vi "yellow_street_vnutr.vi"() -> ()   [LabVIEW 2017]
uses:
  <vilib>/userdefined/High Color/IMAQdx.ctl
  <vilib>/myRIO/Instrument Drivers/Onboard IO/DIO/typedefs/DIO Reference.ctl
  <vilib>/myRIO/Common/Instrument Driver Framework/Utilities/typedefs/myRIO Generic Hardware Reference.ctl
  <vilib>/myRIO/Common/Instrument Driver Framework/Utilities/typedefs/Hardware Version Enum.ctl
  <vilib>/myRIO/Common/Instrument Driver Framework/Utilities/typedefs/myRIO v1.0 Reference.ctl
  <vilib>/myRIO/Common/Instrument Driver Framework/Utilities/typedefs/Generic FPGA Reference.ctl
  <vilib>/myRIO/Common/Instrument Driver Framework/myRIO v1.0/DIO/typedefs/DIO Channels List.ctl
  <vilib>/myRIO/Common/Instrument Driver Framework/myRIO v1.0/DIO/typedefs/DIO Channels Enum.ctl
  <vilib>/userdefined/High Color/nirio_resource_hc.ctl
  <vilib>/myRIO/Common/Instrument Driver Framework/Utilities/vis/Is FPGA Ref Available.vi
  <vilib>/myRIO/Common/Instrument Driver Framework/myRIO v1.0/DIO/vis/myRIO v1.1 Open DIO.vi
  <vilib>/myRIO/Instrument Drivers/Onboard IO/DIO/vis/Write.vi
  <vilib>/myRIO/Common/Instrument Driver Framework/Utilities/vis/Validate Channels.vi
  <vilib>/myRIO/Common/Instrument Driver Framework/myRIO v1.0/DIO/vis/myRIO v1.0 Reserve DIO.vi
  <vilib>/myRIO/Common/Instrument Driver Framework/myRIO v1.0/Resource Manager/vis/myRIO v1.0 Reserve Channel List.vi
  <vilib>/myRIO/Common/Instrument Driver Framework/myRIO v1.0/DIO/vis/myRIO v1.0 Build MUX Configuration DIO.vi
  <vilib>/myRIO/Common/Instrument Driver Framework/myRIO v1.0/Resource Manager/vis/myRIO v1.0 Reserve Channel.vi
  <vilib>/myRIO/Common/Instrument Driver Framework/myRIO v1.0/Resource Manager/vis/myRIO v1.0 Unreserve Channel.vi
  <vilib>/myRIO/Common/Instrument Driver Framework/myRIO v1.0/Resource Manager/vis/myRIO v1.0 Create Configuration List.vi
  <vilib>/myRIO/Common/Instrument Driver Framework/myRIO v1.0/Resource Manager/vis/myRIO v1.0 Build Mutex Name.vi
  <vilib>/Utility/VariantDataType/GetNumericInfo.vi
  <vilib>/Utility/error.llb/Error Cluster From Error Code.vi
  <vilib>/myRIO/Common/Instrument Driver Framework/myRIO v1.0/myRIO v1.1 Open.vi
  <vilib>/myRIO/Common/Instrument Driver Framework/Utilities/vis/IO Manager.vi
  <vilib>/myRIO/Common/Instrument Driver Framework/Utilities/vis/Configuration Manager.vi
  <vilib>/myRIO/Common/Instrument Driver Framework/myRIO v1.0/Resource Manager/vis/myRIO v1.0 Configure IO.vi
  <vilib>/myRIO/Common/Instrument Driver Framework/myRIO v1.0/myRIO v1.0 Close.vi
  <vilib>/myRIO/Common/Instrument Driver Framework/myRIO v1.0/DIO/vis/myRIO v1.0 Write DIO.vi
  <vilib>/myRIO/Express VI/Onboard Devices/LED/LED Express VI.xnode
  <vilib>/myRIO/Instrument Drivers/Onboard IO/DIO/vis/myRIO DIO Open.xnode
  <vilib>/vision/driver/NI_Vision_Acquisition_Software.lvlib
  <vilib>/myRIO/Instrument Drivers/Onboard IO/DIO/DIO.lvlib
panel:
  out "X 4":sgl
  out "X 3":sgl
  out "X 2":sgl
  out "X":sgl
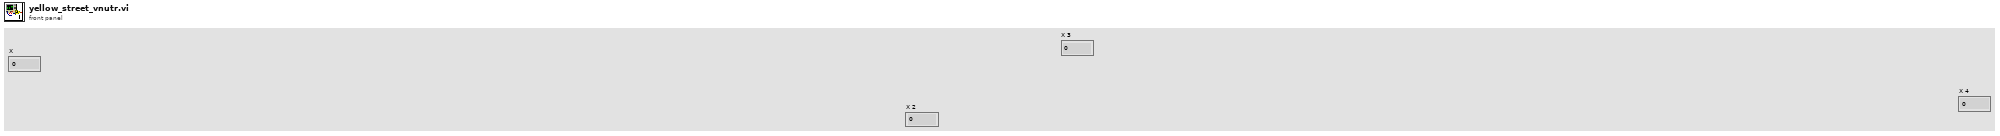
[diagram p1: front panel]
types:
  T1 = typedef "IMAQdx.ctl" = refnum<k21>
  T2 = typedef "DIO.lvlib/DIO Reference.ctl" = cluster{"myRIO Reference":T3, "DIO Channels List":T7}
  T3 = typedef "myRIO Generic Hardware Reference.ctl" = cluster{"myRIO Model":T4, "myRIO Hardware Reference":T5}
  T4 = typedef "Hardware Version Enum.ctl" = enum16{"Unknown", "myRIO-1900", "myRIO-1950", "roboRIO", "NI ELVIS RIO CM"}
  T5 = typedef "myRIO v1.0 Reference.ctl" = cluster{"Generic FPGA Reference":T6, "Allow multiple opens":bool}
  T6 = typedef "Generic FPGA Reference.ctl" = refnum<k20>
  T7 = typedef "DIO Channels List.ctl" = T8[]
  T8 = typedef "DIO Channels Enum.ctl" = enum16{"Not Connected", "C/DIO0", "C/DIO1", "C/DIO2", "C/DIO3", "C/DIO4", "C/DIO5", "C/DIO6", "C/DIO7", "A/DIO0", "A/DIO1", "A/DIO2", "A/DIO3", "A/DIO4", "A/DIO5", "A/DIO6", "A/DIO7", "A/DIO8", "A/DIO9", "A/DIO10", "A/DIO11", "A/DIO12", "A/DIO13", "A/DIO14", "A/DIO15", "B/DIO0", "B/DIO1", "B/DIO2", "B/DIO3", "B/DIO4", "B/DIO5", "B/DIO6", "B/DIO7", "B/DIO8", "B/DIO9", "B/DIO10", "B/DIO11", "B/DIO12", "B/DIO13", "B/DIO14", "B/DIO15", "LED0", "LED1", "LED2", "LED3", "Button0", "DIO/DIO0", "DIO/DIO1", "DIO/DIO2", "DIO/DIO3", "DIO/DIO4", "DIO/DIO5", "DIO/DIO6", "DIO/DIO7", "DIO/DIO8", "DIO/DIO9", "SPI/CS0", "SPI/CS1", "SPI/CS2", "SPI/CS3", "LED RADIO (Green)", "LED RADIO (Red)", "LED COMM (Green)", "LED COMM (Red)", "LED MODE (Green)", "LED MODE (Red)"}
  T9 = typedef "nirio_resource_hc.ctl" = tag
  T10 = typedef "IMAQ Image.ctl" = refnum<image>
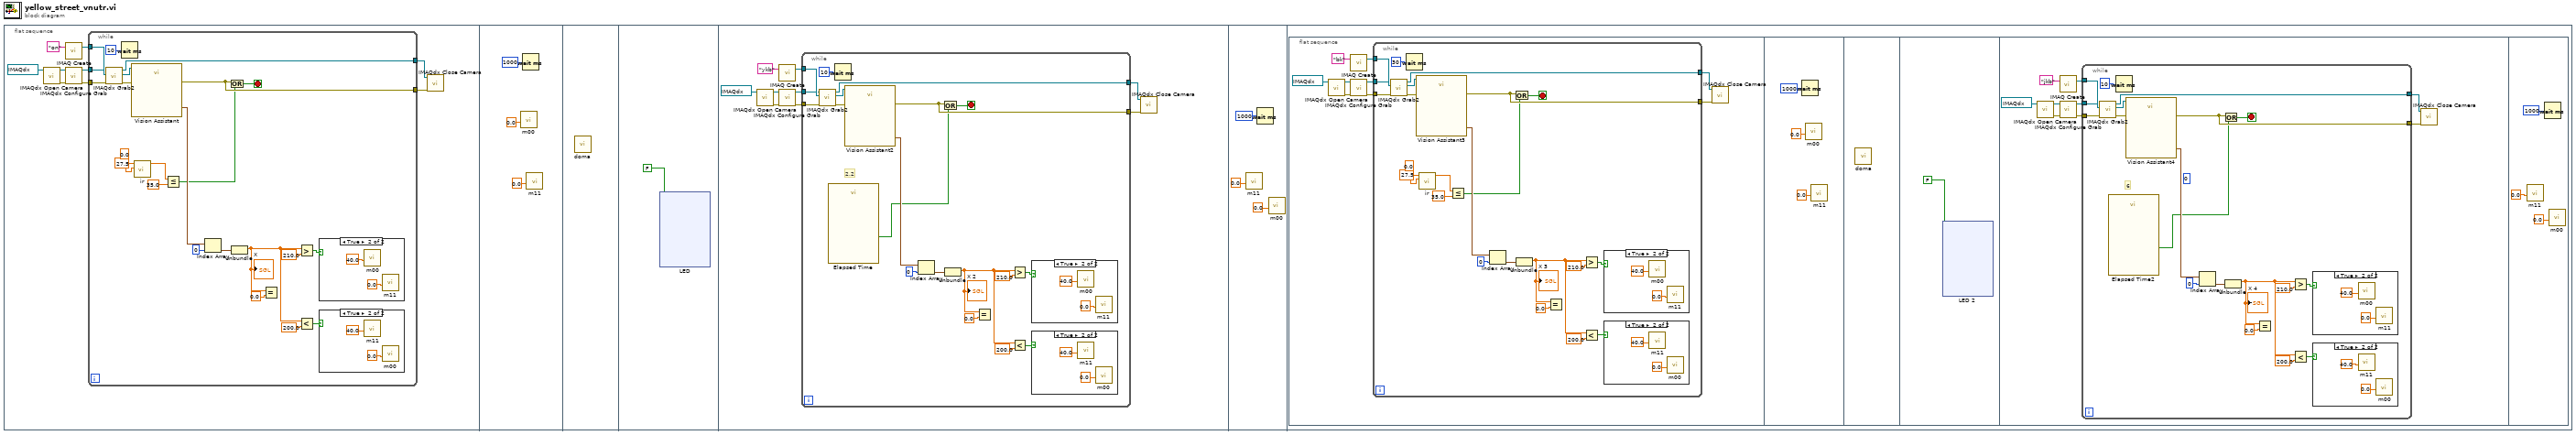
[diagram p0: block diagram]
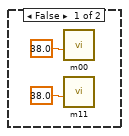
[diagram p2: hidden frame]
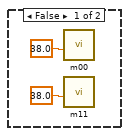
[diagram p3: hidden frame]
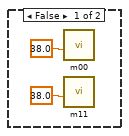
[diagram p4: hidden frame]
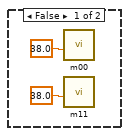
[diagram p5: hidden frame]
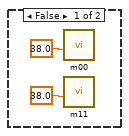
[diagram p6: hidden frame]
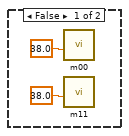
[diagram p7: hidden frame]
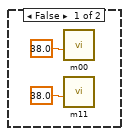
[diagram p8: hidden frame]
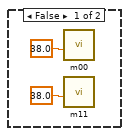
[diagram p9: hidden frame]
diagram:
  n1 = flat-sequence {
    frame #0 {
      n2 = call <vilib>:"IMAQdx Open Camera.vi"("Session In"=T1 "cam1") -> ("error out"=w6:errorcluster, "Session Out"=w5:T1)  [unwired: 9 in]
      n3 = call "IMAQ Create"("Image Name"="on") -> ("New Image"=w3:T10)  [unwired: 4 in, 1 out]
      n4 = call <vilib>:"IMAQdx Configure Grab.vi"("error in"=w6, "Session In"=w5) -> ("error out"=w7:errorcluster, "Session Out"=w4:T1)  [unwired: 8 in]
      n5 = while {
        tunnel: w7 -> [w27]
        tunnel: w3 -> [w26]
        tunnel: w4 -> [w25]
        tunnel: [w24] -> w9
        tunnel: [w23] -> w8
        stop <- w10 stop-if-true
        n6 = call <vilib>:"IMAQdx Grab2.vi"("error in"=w27, "Image In"=w26, "Session In"=w25) -> ("error out"=w29:errorcluster, "Image Out"=w28:T10, "Session Out"=w24:T1)  [unwired: 5 in, 1 out]
        n7 = Wait (ms)(milliseconds to wait=u32 10) -> ()  [unwired: 1 out]
        n8 = call "Vision Assistant"("Image In"=w28, "error in"=w29) -> ("Edges Coordinates (Edge Detector 1)"=w32:cluster{"X":sgl, "Y":sgl}[], "error out"=w23:errorcluster)  [unwired: 22 in, 2 out]
        n9 = call "ir.vi"("Koffset [cm]"=0.0, "Kscale [cm-V]"=27.5) -> ("см"=w15:dbl)  [unwired: 8 in, 1 out]
        n10 = Less Or Equal?(x=w15, y=35.0) -> (x <= y?=w11:bool)
        n11 = Index Array(array=w32, index=0) -> (element=w31:cluster{"X":sgl, "Y":sgl})
        n12 = Or(x=w23, y=w11) -> (x .or. y?=w10:bool)
        n13 = Unbundle(w31) -> ("X"=w18:sgl)  [unwired: 1 out]
        "X" <- w18
        n14 = Equal?(x=w18, y=sgl 0.0) -> ()  [unwired: 1 out]
        n15 = Greater?(x=w18, y=sgl 210.0) -> (0:w21:bool)
        n16 = Less?(x=w18, y=sgl 200.0) -> (x < y?=w17:bool)
        n17 = case shown="True" w21 {
          frame False {
            n18 = call "m00.vi"("position"=38.0) -> ()  [unwired: 10 in, 1 out]
            n19 = call "m11.vi"("position"=38.0) -> ()  [unwired: 10 in, 1 out]
          }
          frame True {
            n20 = call "m00.vi"("position"=40.0) -> ()  [unwired: 10 in, 1 out]
            n21 = call "m11.vi"("position"=0.0) -> ()  [unwired: 10 in, 1 out]
          }
        }
        n22 = case shown="True" w17 {
          frame False {
            n23 = call "m00.vi"("position"=38.0) -> ()  [unwired: 10 in, 1 out]
            n24 = call "m11.vi"("position"=38.0) -> ()  [unwired: 10 in, 1 out]
          }
          frame True {
            n25 = call "m11.vi"("position"=40.0) -> ()  [unwired: 10 in, 1 out]
            n26 = call "m00.vi"("position"=0.0) -> ()  [unwired: 10 in, 1 out]
          }
        }
      }
      n27 = call <vilib>:"IMAQdx Close Camera.vi"("error in"=w8, "Session In"=w9) -> ()  [unwired: 9 in, 1 out]
    }
    frame #1 {
      n28 = call "m00.vi"("position"=0.0) -> ()  [unwired: 10 in, 1 out]
      n29 = Wait (ms)(milliseconds to wait=u32 1000) -> ()  [unwired: 1 out]
      n30 = call "m11.vi"("position"=0.0) -> ()  [unwired: 10 in, 1 out]
    }
    frame #2 {
      n31 = call "doma.vi"() -> ()  [unwired: 12 in]
    }
    frame #3 {
      w44 = FALSE
      n32 = xnode "LED"("LED0"=w44, "LED1"=w44, "LED2"=w44, "LED3"=w44) -> ()  [unwired: 1 in, 1 out]
    }
    frame #4 {
      n33 = call <vilib>:"IMAQdx Open Camera.vi"("Session In"=T1 "cam1") -> ("error out"=w88:errorcluster, "Session Out"=w87:T1)  [unwired: 9 in]
      n34 = call "IMAQ Create"("Image Name"="ykb") -> ("New Image"=w85:T10)  [unwired: 4 in, 1 out]
      n35 = call <vilib>:"IMAQdx Configure Grab.vi"("error in"=w88, "Session In"=w87) -> ("error out"=w89:errorcluster, "Session Out"=w86:T1)  [unwired: 8 in]
      n36 = while {
        tunnel: w89 -> [w105]
        tunnel: w85 -> [w104]
        tunnel: w86 -> [w103]
        tunnel: [w102] -> w91
        tunnel: [w101] -> w90
        stop <- w93 stop-if-true
        # "2,2"
        n37 = call <vilib>:"IMAQdx Grab2.vi"("error in"=w105, "Image In"=w104, "Session In"=w103) -> ("error out"=w107:errorcluster, "Image Out"=w106:T10, "Session Out"=w102:T1)  [unwired: 5 in, 1 out]
        n38 = call "Elapsed Time"() -> ("Time has Elapsed"=w92:bool)  [unwired: 12 in, 7 out]
        n39 = Wait (ms)(milliseconds to wait=u32 10) -> ()  [unwired: 1 out]
        n40 = call "Vision Assistant2"("Image In"=w106, "error in"=w107) -> ("Edges Coordinates (Edge Detector 1)"=w110:cluster{"X":sgl, "Y":sgl}[], "error out"=w101:errorcluster)  [unwired: 22 in, 2 out]
        n41 = Index Array(array=w110, index=0) -> (element=w109:cluster{"X":sgl, "Y":sgl})
        n42 = Or(x=w101, y=w92) -> (x .or. y?=w93:bool)
        n43 = Unbundle(w109) -> ("X"=w96:sgl)  [unwired: 1 out]
        "X 2" <- w96
        n44 = Equal?(x=w96, y=sgl 0.0) -> ()  [unwired: 1 out]
        n45 = Greater?(x=w96, y=sgl 210.0) -> (0:w99:bool)
        n46 = Less?(x=w96, y=sgl 200.0) -> (x < y?=w95:bool)
        n47 = case shown="True" w99 {
          frame False {
            n48 = call "m00.vi"("position"=38.0) -> ()  [unwired: 10 in, 1 out]
            n49 = call "m11.vi"("position"=38.0) -> ()  [unwired: 10 in, 1 out]
          }
          frame True {
            n50 = call "m00.vi"("position"=40.0) -> ()  [unwired: 10 in, 1 out]
            n51 = call "m11.vi"("position"=0.0) -> ()  [unwired: 10 in, 1 out]
          }
        }
        n52 = case shown="True" w95 {
          frame False {
            n53 = call "m00.vi"("position"=38.0) -> ()  [unwired: 10 in, 1 out]
            n54 = call "m11.vi"("position"=38.0) -> ()  [unwired: 10 in, 1 out]
          }
          frame True {
            n55 = call "m11.vi"("position"=40.0) -> ()  [unwired: 10 in, 1 out]
            n56 = call "m00.vi"("position"=0.0) -> ()  [unwired: 10 in, 1 out]
          }
        }
      }
      n57 = call <vilib>:"IMAQdx Close Camera.vi"("error in"=w90, "Session In"=w91) -> ()  [unwired: 9 in, 1 out]
    }
    frame #5 {
      n58 = call "m11.vi"("position"=0.0) -> ()  [unwired: 10 in, 1 out]
      n59 = Wait (ms)(milliseconds to wait=u32 1000) -> ()  [unwired: 1 out]
      n60 = call "m00.vi"("position"=0.0) -> ()  [unwired: 10 in, 1 out]
    }
    frame #6 {
      n61 = flat-sequence {
        frame #0 {
          n62 = call <vilib>:"IMAQdx Open Camera.vi"("Session In"=T1 "cam1") -> ("error out"=w127:errorcluster, "Session Out"=w126:T1)  [unwired: 9 in]
          n63 = call "IMAQ Create"("Image Name"="bk") -> ("New Image"=w124:T10)  [unwired: 4 in, 1 out]
          n64 = call <vilib>:"IMAQdx Configure Grab.vi"("error in"=w127, "Session In"=w126) -> ("error out"=w128:errorcluster, "Session Out"=w125:T1)  [unwired: 8 in]
          n65 = while {
            tunnel: w128 -> [w148]
            tunnel: w124 -> [w147]
            tunnel: w125 -> [w146]
            tunnel: [w145] -> w130
            tunnel: [w144] -> w129
            stop <- w131 stop-if-true
            n66 = call <vilib>:"IMAQdx Grab2.vi"("error in"=w148, "Image In"=w147, "Session In"=w146) -> ("error out"=w150:errorcluster, "Image Out"=w149:T10, "Session Out"=w145:T1)  [unwired: 5 in, 1 out]
            n67 = Wait (ms)(milliseconds to wait=u32 30) -> ()  [unwired: 1 out]
            n68 = call "Vision Assistant3"("Image In"=w149, "error in"=w150) -> ("Edges Coordinates (Edge Detector 1)"=w153:cluster{"X":sgl, "Y":sgl}[], "error out"=w144:errorcluster)  [unwired: 22 in, 2 out]
            n69 = call "ir.vi"("Koffset [cm]"=0.0, "Kscale [cm-V]"=27.5) -> ("см"=w136:dbl)  [unwired: 8 in, 1 out]
            n70 = Less Or Equal?(x=w136, y=35.0) -> (x <= y?=w132:bool)
            n71 = Index Array(array=w153, index=0) -> (element=w152:cluster{"X":sgl, "Y":sgl})
            n72 = Or(x=w144, y=w132) -> (x .or. y?=w131:bool)
            n73 = Unbundle(w152) -> ("X"=w139:sgl)  [unwired: 1 out]
            "X 3" <- w139
            n74 = Equal?(x=w139, y=sgl 0.0) -> ()  [unwired: 1 out]
            n75 = Greater?(x=w139, y=sgl 210.0) -> (0:w142:bool)
            n76 = Less?(x=w139, y=sgl 200.0) -> (x < y?=w138:bool)
            n77 = case shown="True" w142 {
              frame False {
                n78 = call "m00.vi"("position"=38.0) -> ()  [unwired: 10 in, 1 out]
                n79 = call "m11.vi"("position"=38.0) -> ()  [unwired: 10 in, 1 out]
              }
              frame True {
                n80 = call "m00.vi"("position"=40.0) -> ()  [unwired: 10 in, 1 out]
                n81 = call "m11.vi"("position"=0.0) -> ()  [unwired: 10 in, 1 out]
              }
            }
            n82 = case shown="True" w138 {
              frame False {
                n83 = call "m00.vi"("position"=38.0) -> ()  [unwired: 10 in, 1 out]
                n84 = call "m11.vi"("position"=38.0) -> ()  [unwired: 10 in, 1 out]
              }
              frame True {
                n85 = call "m11.vi"("position"=40.0) -> ()  [unwired: 10 in, 1 out]
                n86 = call "m00.vi"("position"=0.0) -> ()  [unwired: 10 in, 1 out]
              }
            }
          }
          n87 = call <vilib>:"IMAQdx Close Camera.vi"("error in"=w129, "Session In"=w130) -> ()  [unwired: 9 in, 1 out]
        }
        frame #1 {
          n88 = Wait (ms)(milliseconds to wait=u32 1000) -> ()  [unwired: 1 out]
          n89 = call "m00.vi"("position"=0.0) -> ()  [unwired: 10 in, 1 out]
          n90 = call "m11.vi"("position"=0.0) -> ()  [unwired: 10 in, 1 out]
        }
        frame #2 {
          n91 = call "doma.vi"() -> ()  [unwired: 12 in]
        }
        frame #3 {
          w165 = FALSE
          n92 = xnode "LED 2"("LED0"=w165, "LED1"=w165, "LED2"=w165, "LED3"=w165) -> ()  [unwired: 1 in, 1 out]
        }
        frame #4 {
          n93 = call <vilib>:"IMAQdx Open Camera.vi"("Session In"=T1 "cam1") -> ("error out"=w209:errorcluster, "Session Out"=w208:T1)  [unwired: 9 in]
          n94 = call "IMAQ Create"("Image Name"="jkb") -> ("New Image"=w206:T10)  [unwired: 4 in, 1 out]
          n95 = call <vilib>:"IMAQdx Configure Grab.vi"("error in"=w209, "Session In"=w208) -> ("error out"=w210:errorcluster, "Session Out"=w207:T1)  [unwired: 8 in]
          n96 = while {
            tunnel: w210 -> [w226]
            tunnel: w206 -> [w225]
            tunnel: w207 -> [w224]
            tunnel: [w223] -> w212
            tunnel: [w222] -> w211
            stop <- w214 stop-if-true
            (unwired) 0 ("index")
            # "6"
            n97 = call <vilib>:"IMAQdx Grab2.vi"("error in"=w226, "Image In"=w225, "Session In"=w224) -> ("error out"=w228:errorcluster, "Image Out"=w227:T10, "Session Out"=w223:T1)  [unwired: 5 in, 1 out]
            n98 = call "Elapsed Time2"() -> ("Time has Elapsed"=w213:bool)  [unwired: 12 in, 7 out]
            n99 = Wait (ms)(milliseconds to wait=u32 10) -> ()  [unwired: 1 out]
            n100 = call "Vision Assistant4"("Image In"=w227, "error in"=w228) -> ("Edges Coordinates (Edge Detector 1)"=w231:cluster{"X":sgl, "Y":sgl}[], "error out"=w222:errorcluster)  [unwired: 22 in, 2 out]
            n101 = Index Array(array=w231, index=0) -> (element=w230:cluster{"X":sgl, "Y":sgl})
            n102 = Or(x=w222, y=w213) -> (x .or. y?=w214:bool)
            n103 = Unbundle(w230) -> ("X"=w217:sgl)  [unwired: 1 out]
            "X 4" <- w217
            n104 = Equal?(x=w217, y=sgl 0.0) -> ()  [unwired: 1 out]
            n105 = Greater?(x=w217, y=sgl 210.0) -> (0:w220:bool)
            n106 = Less?(x=w217, y=sgl 200.0) -> (x < y?=w216:bool)
            n107 = case shown="True" w220 {
              frame False {
                n108 = call "m00.vi"("position"=38.0) -> ()  [unwired: 10 in, 1 out]
                n109 = call "m11.vi"("position"=38.0) -> ()  [unwired: 10 in, 1 out]
              }
              frame True {
                n110 = call "m00.vi"("position"=40.0) -> ()  [unwired: 10 in, 1 out]
                n111 = call "m11.vi"("position"=0.0) -> ()  [unwired: 10 in, 1 out]
              }
            }
            n112 = case shown="True" w216 {
              frame False {
                n113 = call "m00.vi"("position"=38.0) -> ()  [unwired: 10 in, 1 out]
                n114 = call "m11.vi"("position"=38.0) -> ()  [unwired: 10 in, 1 out]
              }
              frame True {
                n115 = call "m11.vi"("position"=40.0) -> ()  [unwired: 10 in, 1 out]
                n116 = call "m00.vi"("position"=0.0) -> ()  [unwired: 10 in, 1 out]
              }
            }
          }
          n117 = call <vilib>:"IMAQdx Close Camera.vi"("error in"=w211, "Session In"=w212) -> ()  [unwired: 9 in, 1 out]
        }
        frame #5 {
          n118 = call "m11.vi"("position"=0.0) -> ()  [unwired: 10 in, 1 out]
          n119 = Wait (ms)(milliseconds to wait=u32 1000) -> ()  [unwired: 1 out]
          n120 = call "m00.vi"("position"=0.0) -> ()  [unwired: 10 in, 1 out]
        }
      }
    }
  }
